vi "Close connection if open.vi"(0 "System no.":i32=1 min=1 step=1, 2 "Close DaisyChain":bool, 5 "error in":errorcluster) -> (14 "Was connected?":bool, 19 "error out":errorcluster)   [LabVIEW 2020]
doc: "This VI checks if the connection to the selected system is already open and, if it is, it closes this connection."
uses:
  Available interfaces.ctl
  Available DLLs.ctl
  Global1.vi
  Global DaisyChain.vi
panel:
  out "DLL for Device":T1=17 items=["C-843", "C-844", "E-710", "C-843.PM", "C-865", "E-761", "Mercury", "E-755", "E-753", "C-866", "E-712", "E-725", "E-861", "C-867", "E-517", "E-816", "E-709", "PI_GCS2_DLL", "HydraPollux"]
  out "Interface":T2 items=["RS232", "GPIB", "DLL", "TCP-IP", "USB", "Analog"]
  out "VISA resource name":refnum<visa-resource-name>
  # "This vi checks if the connection to the selected system\nis already open and, if it is, it closes this connection."
  # "Communication setup indicators (for troubleshooting):"
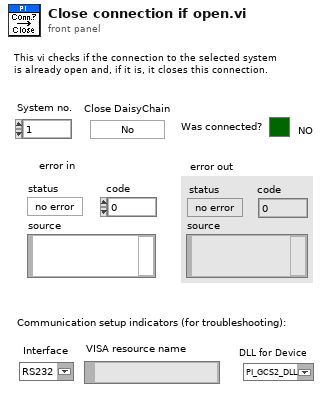
[diagram p1: front panel]
types:
  T1 = typedef "Available DLLs.ctl" = u16
  T2 = typedef "Available interfaces.ctl" = u16
  T3 = cluster{"RS232 Portnumber":i32, "Timeout":i32, "RS232 Baud rate":u32, "Interface":T2, "GPIB Bus":i32, "GPIB Address":i32, "GPIB Mode":i32}[]
  T4 = typedef "Available DLL interfaces.ctl" = u16
  T5 = cluster{"DLL for Device":T1, "DLL Interface":T4, "Parameter":string}[]
  T6 = cluster{"RS232 Portnumber":i32, "Timeout":i32, "RS232 Baud rate":u32, "Interface":T2, "GPIB Bus":i32, "GPIB Address":i32, "GPIB Mode":i32}
  T7 = cluster{"DLL for Device":T1, "DLL Interface":T4, "Parameter":string}
  T8 = enum16{"C844_IsDLLAvailable", "C844_ConnectRS232", "C844_ConnectNIgpib", "C844_IsConnected", "C844_CloseConnection", "C844_GcsCommandset", "C844_GetError", "C844_GcsGetAnswerSize", "C844_GcsGetAnswer", "C843_IsDLLAvailable", "C843_Connect", "C843_IsConnected", "C843_CloseConnection", "C843_GcsCommandset", "C843_GetError", "C843_GcsGetAnswerSize", "C843_GcsGetAnswer", "E710_IsDLLAvailable", "E710_ConnectRS232", "E710_ConnectNIgpib", "E710_IsConnected", "E710_CloseConnection", "E710_GcsCommandset", "E710_GetError", "E710_GcsGetAnswerSize", "E710_GcsGetAnswer", "C843_PM_IsDLLAvailable", "C843_PM_Connect", "C843_PM_IsConnected", "C843_PM_CloseConnection", "C843_PM_GcsCommandset", "C843_PM_GetError", "C843_PM_GcsGetAnswerSize", "C843_PM_GcsGetAnswer", "C843_PM_GetCurrentBoardID", "C843_GetCurrentBoardID", "C865_IsDLLAvailable", "C865_ConnectRS232", "C865_IsConnected", "C865_CloseConnection", "C865_GcsCommandset", "C865_GetError", "C865_GcsGetAnswerSize", "C865_GcsGetAnswer", "C865_GetCurrentInterfaceID", "E761_ConnectPciBoard", "DefineSystem", "CloseConnection", "IsConnected", "ConnectRS232", "ConnectNIgpib", "ConnectPciBoard", "ConnectTCPIP", "GetError", "GcsCommandset", "GCSGetAnswerSize", "GcsGetAnswer"}
  T9 = enum16{"C844_IsDLLAvailable", "C844_ConnectRS232", "C844_ConnectNIgpib", "C844_IsConnected", "C844_CloseConnection", "C844_GcsCommandset", "C844_GetError", "C844_GcsGetAnswerSize", "C844_GcsGetAnswer", "C843_IsDLLAvailable", "C843_Connect", "C843_IsConnected", "C843_CloseConnection", "C843_GcsCommandset", "C843_GetError", "C843_GcsGetAnswerSize", "C843_GcsGetAnswer", "E710_IsDLLAvailable", "E710_ConnectRS232", "E710_ConnectNIgpib", "E710_IsConnected", "E710_CloseConnection", "E710_GcsCommandset", "E710_GetError", "E710_GcsGetAnswerSize", "E710_GcsGetAnswer", "C843_PM_IsDLLAvailable", "C843_PM_Connect", "C843_PM_IsConnected", "C843_PM_CloseConnection", "C843_PM_GcsCommandset", "C843_PM_GetError", "C843_PM_GcsGetAnswerSize", "C843_PM_GcsGetAnswer", "C843_PM_GetCurrentBoardID", "C843_GetCurrentBoardID", "C865_IsDLLAvailable", "C865_ConnectRS232", "C865_IsConnected", "C865_CloseConnection", "C865_GcsCommandset", "C865_GetError", "C865_GcsGetAnswerSize", "C865_GcsGetAnswer", "C865_GetCurrentInterfaceID", "E761_ConnectPciBoard", "DefineSystem", "CloseConnection", "IsConnected", "ConnectRS232", "ConnectNIgpib", "ConnectPciBoard", "ConnectTCPIP", "GetError", "GcsCommandset", "GCSGetAnswerSize", "GcsGetAnswer", "CloseDaisyChain", "OpenRS232DaisyChain", "ConnectDaisyChainDevice"}
  T10 = cluster{"No. of devices":i32, "Port ID":i32, "Devices":string[], "Description":string}[]
  T11 = cluster{"No. of devices":i32, "Port ID":i32, "Devices":string[], "Description":string}
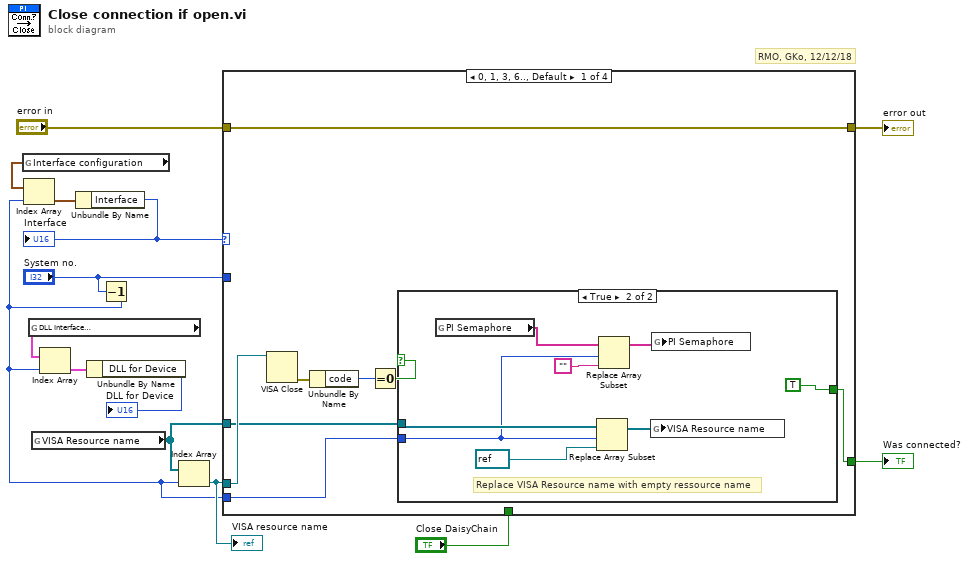
[diagram p0: block diagram]
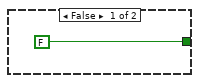
[diagram p2: hidden frame]
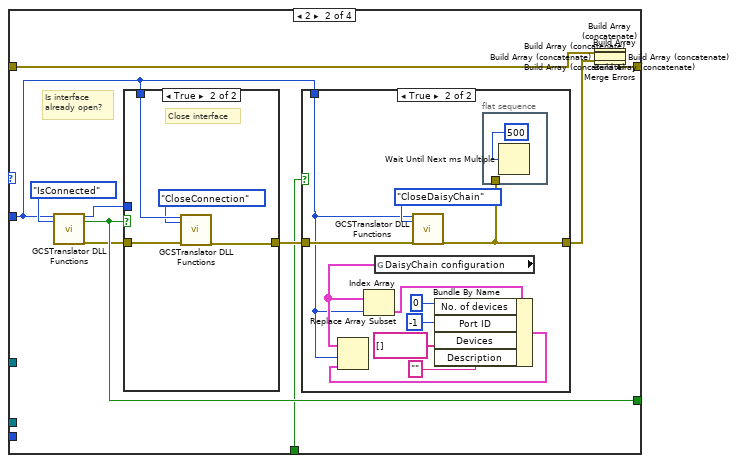
[diagram p3: hidden frame]
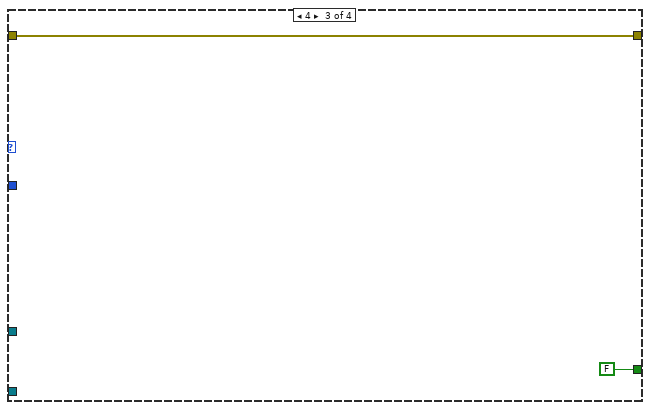
[diagram p6: hidden frame]
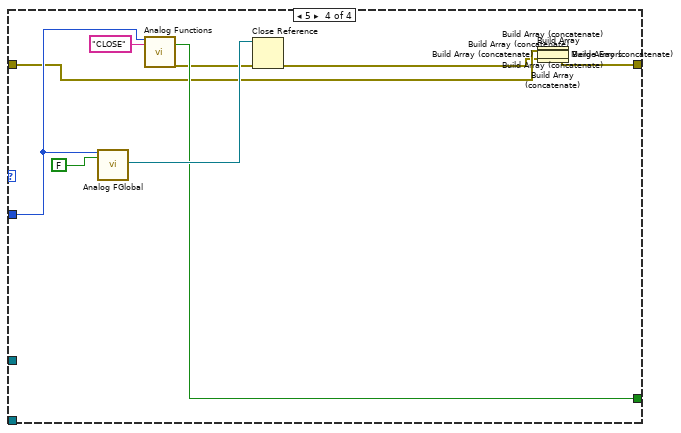
[diagram p7: hidden frame]
diagram:
  # "RMO, GKo, 12/12/18"
  n1 = global read "Global1.vi" "Interface configuration"() -> (w11:T3)
  n2 = global read "Global1.vi" "DLL Interface\nConfiguration"() -> (w4:T5)
  n3 = global read "Global1.vi" "VISA Resource name"() -> (w2:refnum<visa-resource-name>[])
  n4 = Decrement(x="System no.") -> (x-1=w1:i32)
  n5 = Index Array(array=w11, index=w1) -> (element=w10:T6)
  n6 = Index Array(array=w4, index=w1) -> (element=w5:T7)
  n7 = Unbundle By Name(w10) -> ("Interface"=w7:T2)
  "Interface" <- w7
  n8 = Unbundle By Name(w5) -> ("DLL for Device"=→"DLL for Device":T1)
  n9 = Index Array(array=w2, index=w1) -> (element=w8:refnum<visa-resource-name>)
  "VISA resource name" <- w8
  n10 = case shown="0, 1, 3, 6.., Default" w7 {
    tunnel: "error in" -> [w21 w40 w68 w77]
    tunnel: [w21 w41 w68 w78] -> w13
    tunnel: "System no." -> [_ w42 _ w82]
    tunnel: [w20 w48 FALSE ("Boolean output") w80] -> w12
    tunnel: w8 -> [w22 _ _ _]
    tunnel: "Close DaisyChain" -> [_ w43 _ _]
    tunnel: w2 -> [w16 _ _ _]
    tunnel: w1 -> [w15 _ _ _]
    frame 0, 1, 3, 6.., Default {
      n11 = VISA Close(VISA resource name=w22) -> (error out=w19:errorcluster)  [unwired: 1 in]
      n12 = Unbundle By Name(w19) -> ("code"=w18:i32)
      n13 = Equal To 0?(x=w18) -> (x = 0?=w17:bool)
      n14 = case shown="True" w17 {
        tunnel: [FALSE ("Boolean output") TRUE ("Boolean output")] -> w20
        tunnel: w16 -> [_ w30]
        tunnel: w15 -> [_ w24]
        frame False {
        }
        frame True {
          # "Replace VISA Resource name with empty ressource name"
          n15 = global read "Global1.vi" "PI Semaphore"() -> (w27:string[])
          n16 = Replace Array Subset(array=w30, new element=refnum<visa-resource-name> refnum ("new element/subarray"), index=w24) -> (w28:refnum<visa-resource-name>[])
          n17 = Replace Array Subset(array=w27, new element="", index=w24) -> (w26:string[])
          n18 = global write "Global1.vi" "VISA Resource name"(w28) -> ()
          n19 = global write "Global1.vi" "PI Semaphore"(w26) -> ()
        }
      }
    }
    frame 2 {
      # "Is interface\nalready open?"
      n20 = call "GCSTranslator DLL Functions.vi"("System no."=w42, "Function"=T8."IsConnected") -> ("DLL I32 Return value"=w46:i32, "Boolean output"=w48:bool, "error out"=w47:errorcluster)  [unwired: 5 in, 10 out]
      n21 = case shown="True" w48 {
        tunnel: w47 -> [w62 w66]
        tunnel: [w62 w65] -> w44
        tunnel: w42 -> [_ w64]
        tunnel: w46 -> [_ _]
        frame False {
        }
        frame True {
          # "Close interface"
          n22 = call "GCSTranslator DLL Functions.vi"("System no."=w64, "Function"=T8."CloseConnection", "error in"=w66) -> ("error out"=w65:errorcluster)  [unwired: 4 in, 12 out]
        }
      }
      n23 = case shown="True" w43 {
        tunnel: w44 -> [w49 w59]
        tunnel: [w49 w58] -> w39
        tunnel: w42 -> [_ w50]
        frame False {
        }
        frame True {
          n24 = global read "Global DaisyChain.vi" "DaisyChain configuration"() -> (w56:T10)
          n25 = Index Array(array=w56, index=w50) -> (element=w51:T11)
          n26 = call "GCSTranslator DLL Functions.vi"("System no."=w50, "Function"=T9."CloseDaisyChain", "error in"=w59) -> ("error out"=w58:errorcluster)  [unwired: 4 in, 12 out]
          n27 = Bundle By Name(cluster=w51, "No. of devices"=0, "Port ID"=-1, "Devices"=string[] [], "Description"="") -> (w57:T11)
          n28 = Replace Array Subset(array=w56, new element=w57, index=w50) -> ()  [unwired: 1 out]
          n29 = flat-sequence {
            tunnel: w58 -> [_]
            frame #0 {
              n30 = Wait Until Next ms Multiple(millisecond multiple=u32 500) -> ()  [unwired: 1 out]
            }
          }
        }
      }
      n31 = Build Array(w40, w39) -> (w38:errorcluster[])
      n32 = Build Array (concatenate)(w38) -> (w37:errorcluster[])
      n33 = Build Array (concatenate)(w37) -> (w36:errorcluster[])
      n34 = Build Array (concatenate)(w36) -> (w35:errorcluster[])
      n35 = Build Array (concatenate)(w35) -> (w34:errorcluster[])
      n36 = Build Array (concatenate)(w34) -> (w33:errorcluster[])
      n37 = Build Array (concatenate)(w33) -> (w32:errorcluster[])
      n38 = Merge Errors(w32) -> (w41:errorcluster)
    }
    frame 4 {
    }
    frame 5 {
      n39 = call "Analog FGlobal.vi"("System no."=w82, "Read(F)/Write"=FALSE) -> ("VI ref out"=w83:refnum<vi>)  [unwired: 1 in, 16 out]
      n40 = call "Analog Functions.vi"("System no."=w82, "String to send"="CLOSE") -> ("Boolean output"=w80:bool, "error out"=w79:errorcluster)  [unwired: 5 in, 11 out]
      n41 = Close Reference(reference=w83, error in (no error)=w79) -> (error out=w76:errorcluster)
      n42 = Build Array(w77, w76) -> (w75:errorcluster[])
      n43 = Build Array (concatenate)(w75) -> (w74:errorcluster[])
      n44 = Build Array (concatenate)(w74) -> (w73:errorcluster[])
      n45 = Build Array (concatenate)(w73) -> (w72:errorcluster[])
      n46 = Build Array (concatenate)(w72) -> (w71:errorcluster[])
      n47 = Build Array (concatenate)(w71) -> (w70:errorcluster[])
      n48 = Build Array (concatenate)(w70) -> (w69:errorcluster[])
      n49 = Merge Errors(w69) -> (w78:errorcluster)
    }
  }
  "error out" <- w13
  "Was connected?" <- w12
